vi "ULx Write (Digital 1D Wfm NChan NSamp).vi"(0 "task in":refnum<k24>, 1 "auto start":bool, 7 "data":digitalwaveform[](array[waveform]), 9 "timeout":dbl=10.0 format="%_4g", 11 "error in":errorcluster) -> (4 "task out":refnum<k24>, 10 "number of samples written per channel":u32, 15 "error out":errorcluster)   [LabVIEW 2020]
doc: "Writes one or more digital waveforms to a task that contains one or more digital output channels."
uses:
  C:/Users/William/Documents/LV 2020 builds/LeaktestDAQ/Source-v33/ULx_LV.dll
  ULx_LV.dll
panel:
  # "channel"
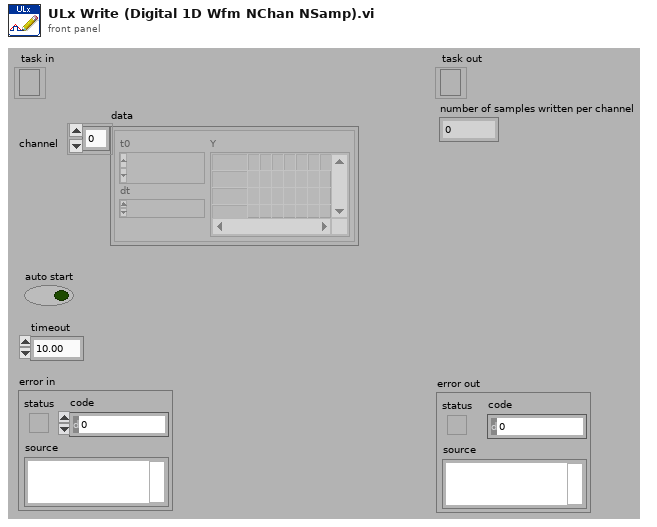
[diagram p1: front panel]
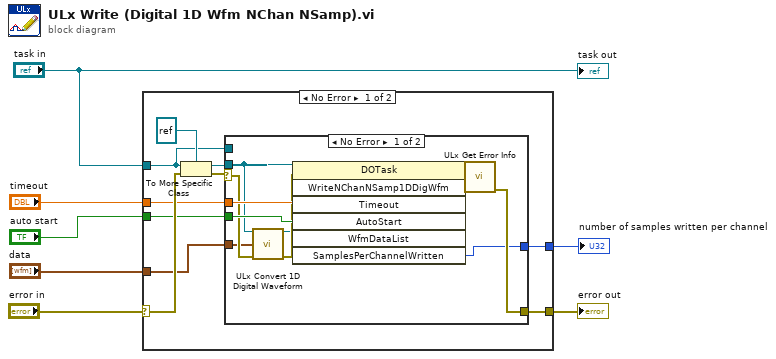
[diagram p0: block diagram]
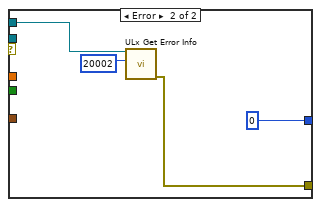
[diagram p2: hidden frame]
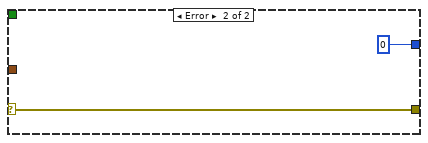
[diagram p3: hidden frame]
diagram:
  n1 = case shown="No Error" "error in" {
    selector: "error in" -> [w17 w35]
    tunnel: "task in" -> [w11 _]
    tunnel: "timeout" -> [w13 _]
    tunnel: [w12 w35] -> w5
    tunnel: "auto start" -> [w10 _]
    tunnel: [w9 0 ("SamplesPerChannelWritten")] -> w2
    tunnel: "data" -> [w8 _]
    frame No Error {
      n2 = To More Specific Class(target class=refnum<k24> refnum, reference=w11, error in=w17) -> (specific class reference=w14:refnum<k24>, error out=w15:errorcluster)
      n3 = case shown="No Error" w15 {
        selector: w15 -> [w22 _]
        tunnel: w14 -> [w20 _]
        tunnel: w13 -> [w24 _]
        tunnel: [w27 w32] -> w12
        tunnel: w11 -> [_ w31]
        tunnel: w10 -> [w23 _]
        tunnel: [w25 0 ("SamplesPerChannelWritten")] -> w9
        tunnel: w8 -> [w19 _]
        frame No Error {
          n4 = call "ULx Convert 1D Digital Waveform.vi"("task in"=w20, "data"=w19, "error in"=w22) -> ("data List"=w18:refnum<k24>, "error out"=w21:errorcluster)  [unwired: 11 in]
          n5 = invoke class="DOTask" method="WriteNChanNSamp1DDigWfm"(reference=w20, error in=w21, "Timeout"=w24, "AutoStart"=w23, "WfmDataList"=w18) -> (reference out=w28:refnum<k24>, error out=w29:errorcluster, "WriteNChanNSamp1DDigWfm"=w26:i32, "SamplesPerChannelWritten"=w25:u32)  [unwired: 2 in, 3 out]
          n6 = call "ULx Get Error Info.vi"("error in"=w29, "ErrorCode"=w26, "task in"=w28) -> ("error out"=w27:errorcluster)  [unwired: 8 in]
        }
        frame Error {
          n7 = call "ULx Get Error Info.vi"("ErrorCode"=20002, "task in"=w31) -> ("error out"=w32:errorcluster)  [unwired: 9 in]
        }
      }
    }
    frame Error {
    }
  }
  "error out" <- w5
  "number of samples written per channel" <- w2
  "task out" <- "task in"
